vi "Calibrate NART DUT.vi"(0 "RFSA Device":refnum<k15>="RFSA" caption="instrument handle", 1 "port":u16=3363, 2 "Host":string="10.234.39.192", 3 "CART TCP Connection In":refnum<k5>, 5 "Measurement Handle In":T3, 7 "Frequency and Tx Gain":T4[](array[typedef]), 11 "error in (no error)":errorcluster, 12 "Path Loss, dB":dbl[][](array[numeric]) format="%.2f", 13 "Measurement Timeout, sec":T1=10.0 format="%.3f") -> (4 "RFSA Handle Out":T2="RFSA" caption="RFSA Handle", 6 "Measurement Handle Out":T3, 8 "CART TCP Connection Out":refnum<k5>, 15 "error out":errorcluster)   [LabVIEW 2011]
uses:
  LVx Folder/Support/TypeDef/TX Cal Data Rate.ctl
  <userlib>/niRF/niBasic/SA/Waveform/Includes/niBASIC - SA - Waveform - INC - STYP - Measurement Handle.ctl
  <userlib>/niRF/niBasic/SA/Waveform/Includes/niBASIC - SA - Waveform - INC - STYP - State Element.ctl
  <userlib>/niRF/niSystem/SA/Includes/niSYS - SA - INC - STYP - Measurement Interval.ctl
  <userlib>/niRF/niSystem/SA/Includes/niSYS - SA - INC - STYP - RBW Filter.ctl
  <userlib>/niRF/niSystem/SA/Includes/niSYS - SA - INC - STYP - External Attenuation.ctl
  <userlib>/niRF/niBasic/SA/Waveform/Includes/niBASIC - SA - Waveform - INC - STYP - Averaging.ctl
  <userlib>/niRF/niSystem/SA/Includes/niSYS - RFSA - INC - STYP - Handle.ctl
  <userlib>/niRF/niSystem/SA/Includes/niSYS - SA - INC - STYP - Timeout.ctl
  <userlib>/niRF/niSystem/SA/Includes/niSYS - SA - INC - STYP - Measurement Request.ctl
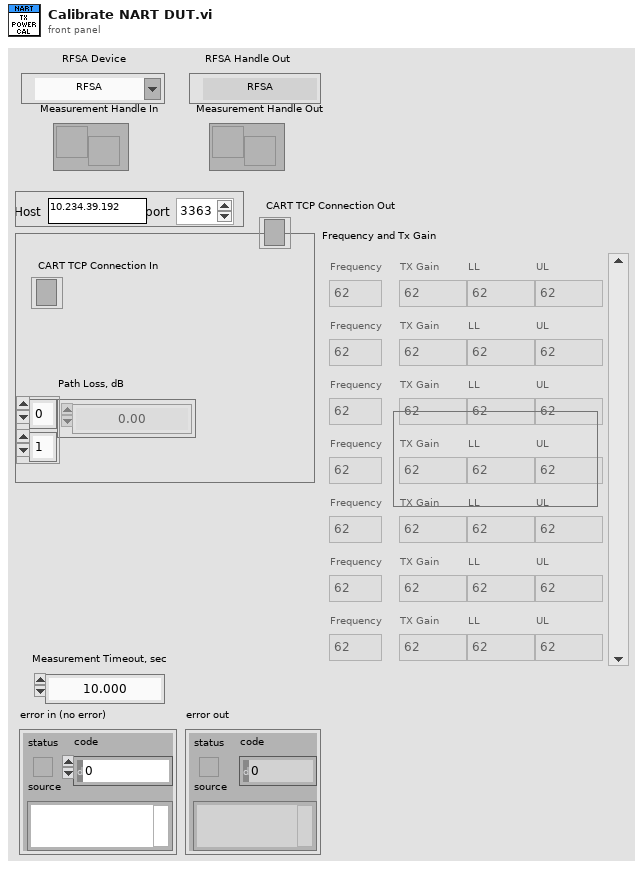
[diagram p1: front panel]
types:
  T1 = typedef "niSYS - SA - INC - STYP - Timeout.ctl" = dbl
  T2 = typedef "niSYS - RFSA - INC - STYP - Handle.ctl" = refnum<k15>
  T3 = typedef "niBASIC - SA - Waveform - INC - STYP - Measurement Handle.ctl" = refnum<notifier>
  T4 = typedef "TX Cal Data Rate.ctl" = cluster{"Frequency":u32, "TX Gain":u32, "LL":i32, "UL":u32}
  T5 = typedef "niSYS - SA - INC - STYP - Measurement Interval.ctl" = dbl
  T6 = typedef "niSYS - SA - INC - STYP - Measurement Request.ctl" = enum16{"Measure", "Fetch", "Initiate"}
  T7 = cluster{"Frequency, MHz":u32, "TX Gain":u32, "Data Rate":string, "Packet Length":u32, "Packet Count":i32}
  T8 = typedef "niBASIC - SA - Waveform - INC - STYP - Measurement.ctl" = cluster{"Mean Power, dBm":dbl, "Peak to Average Ratio, dB":dbl, "Maximum Power, dBm":dbl, "Minimum Power, dBm":dbl}
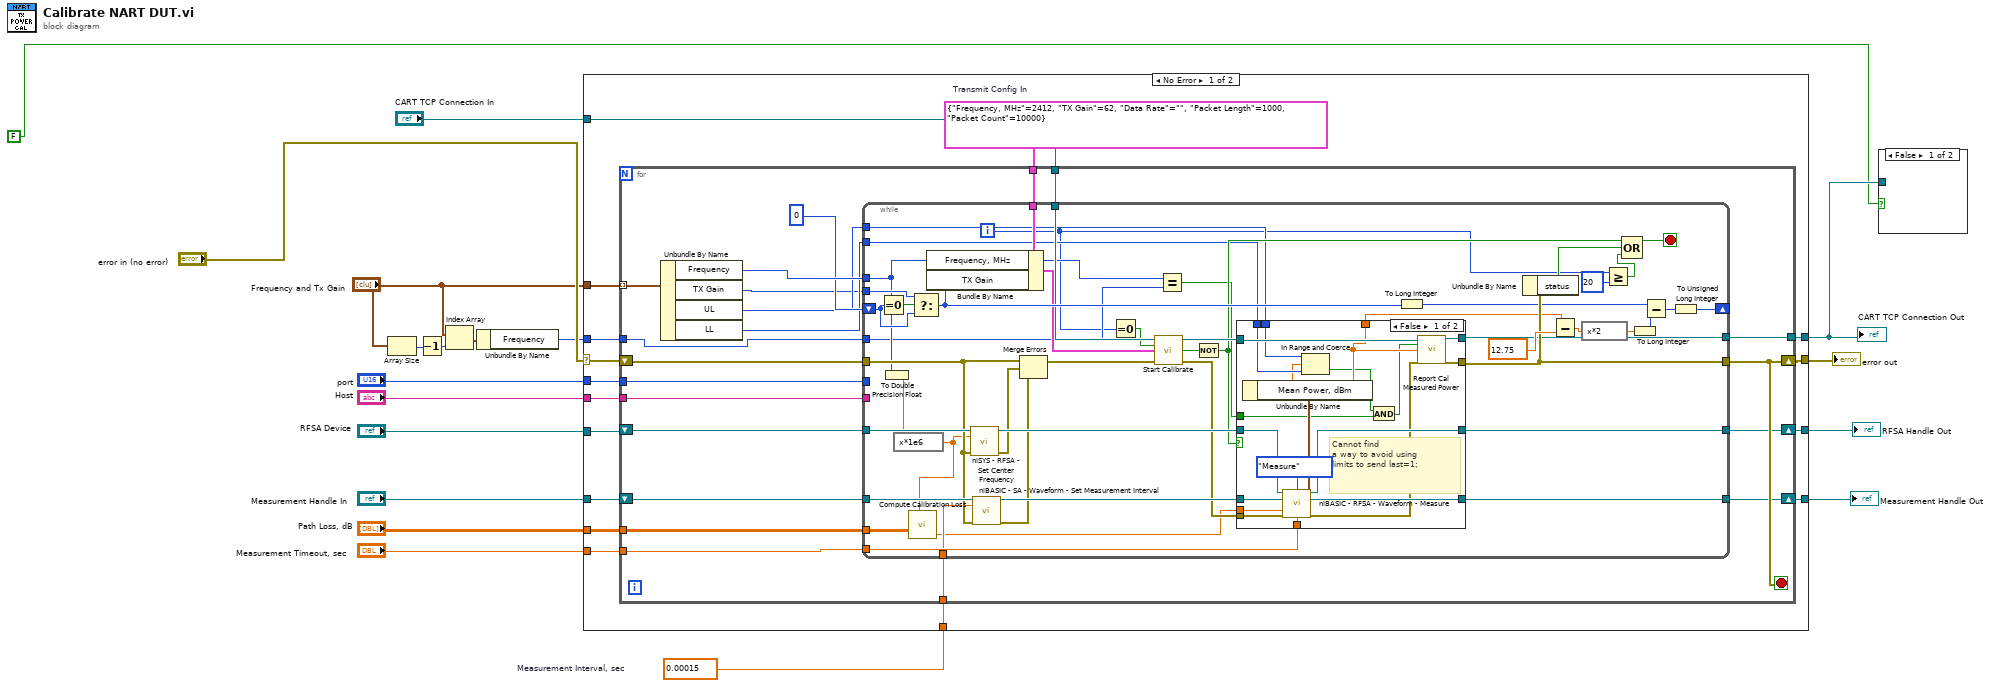
[diagram p0: block diagram]
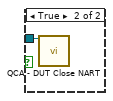
[diagram p2: hidden frame]
diagram:
  w11 = T5 0.00015  # Measurement Interval, sec
  n1 = Array Size(array="Frequency and Tx Gain") -> (size(s)=w4:i32)
  n2 = Decrement(x=w4) -> (x-1=w3:i32)
  n3 = Index Array(array="Frequency and Tx Gain", index=w3) -> (element=w2:T4)
  n4 = Unbundle By Name(w2) -> ("Frequency"=w1:u32)
  n5 = case shown="No Error" "error in (no error)" {
    selector: "error in (no error)" -> [w33 w131]
    tunnel: [w22 w131] -> w17
    tunnel: "port" -> [w21 _]
    tunnel: "Host" -> [w32 _]
    tunnel: "Frequency and Tx Gain" -> [w34 _]
    tunnel: "Measurement Handle In" -> [w31 w129]
    tunnel: [w30 w129] -> w15
    tunnel: "RFSA Device" -> [w29 w130]
    tunnel: [w28 w130] -> w13
    tunnel: "Path Loss, dB" -> [w27 _]
    tunnel: "Measurement Timeout, sec" -> [w26 _]
    tunnel: w11 -> [w25 _]
    tunnel: "CART TCP Connection In" -> [w24 w128]
    tunnel: [w20 w128] -> w9
    tunnel: w1 -> [w23 _]
    frame No Error {
      w35 = T7 {"Frequency, MHz"=2412, "TX Gain"=62, "Data Rate"="", "Packet Length"=1000, "Packet Count"=10000}  # Transmit Config In
      n6 = for {
        tunnel: w21 -> [w56]
        tunnel: w32 -> [w55]
        tunnel: w35 -> [w54]
        tunnel: w34 -> [w53] mode=indexing
        shift-right: [w52] -> w22
        shift-left: w33 -> [w51]
        shift-right: [w49] -> w30
        shift-left: w31 -> [w50]
        shift-right: [w47] -> w28
        shift-left: w29 -> [w48]
        tunnel: w27 -> [w46]
        tunnel: w26 -> [w45]
        tunnel: w25 -> [w44]
        tunnel: w24 -> [w43]
        tunnel: [w42] -> w20
        tunnel: w23 -> [w41]
        stop <- w52 stop-if-true
        n7 = Unbundle By Name(w53) -> ("Frequency"=w40:u32, "TX Gain"=w36:u32, "UL"=w38:u32, "LL"=w37:i32)
        n8 = while {
          tunnel: w54 -> [w104]
          tunnel: w56 -> [_]
          tunnel: [w78] -> w52
          tunnel: w55 -> [_]
          tunnel: w50 -> [w102]
          tunnel: [w101] -> w49
          tunnel: [w100] -> w47
          tunnel: w46 -> [w71]
          tunnel: w45 -> [w99]
          tunnel: w48 -> [w98]
          tunnel: w40 -> [w67]
          tunnel: w51 -> [w96]
          tunnel: w44 -> [w93]
          shift-right: [w84] -> _
          shift-left: u32 0 ("TX Gain") -> [w88]
          tunnel: w36 -> [w91]
          tunnel: w43 -> [w74]
          tunnel: [w72] -> w42
          tunnel: w38 -> [w62]
          tunnel: w37 -> [w61]
          tunnel: w41 -> [w66]
          i -> [w58]
          stop <- w83 stop-if-true
          n9 = Equal To 0?(x=w88) -> (x = 0?=w92:bool)
          n10 = To Double Precision Float(number=w67) -> (double precision float=w81:dbl)
          n11 = expression code="x*1e6"(w81) -> (w70:dbl)
          n12 = call "Compute Calibration Loss.vi"("Table (frequency, power, pathloss)"=w71, "Center Frequency, Hz"=w70) -> ("External Attenuation, dB"=w69:dbl)  [unwired: 3 in, 2 out]
          n13 = Select(t=w91, s=w92, f=w88) -> (s? t:f=w87:u32)
          n14 = Bundle By Name(cluster=w104, "Frequency, MHz"=w67, "TX Gain"=w87) -> (w75:T7)
          n15 = call <userlib>:"niSYS - RFSA - Set Center Frequency.vi"("RFSA Handle In"=w98, "RFSA Center Frequency, Hz"=w70, "error in (no error)"=w96) -> ("RFSA Handle Out"=w97:T2, "error out"=w95:errorcluster)  [unwired: 11 out]
          n16 = call <userlib>:"niBASIC - SA - Waveform - Set Measurement Interval.vi"("Measurement Handle In"=w102, "Measurement Interval, sec"=w93, "error in (no error)"=w96) -> ("Measurement Handle Out"=w103:T3, "error out"=w94:errorcluster)  [unwired: 11 out]
          n17 = Merge Errors(w96, w95, w94) -> (w76:errorcluster)
          n18 = Equal To 0?(x=w58) -> (x = 0?=w68:bool)
          n19 = call "Start Calibrate.vi"("CART TCP Connection In"=w74, "Send Cal Command?"=w68, "Calibrate Config"=w75, "error in (no error)"=w76) -> ("CART TCP Connection Out"=w73:refnum<k5>, "More Pwr Reporting?"=w64:bool, "error out"=w77:errorcluster)  [unwired: 7 in, 2 out]
          n20 = Equal?(x=w67, y=w66) -> (x = y?=w63:bool)
          n21 = Not(x=w64) -> (.not. x?=w65:bool)
          n22 = case shown="False" w65 {
            tunnel: w103 -> [w121 w126]
            tunnel: [w120 w126] -> w101
            tunnel: [w119 w127] -> w100
            tunnel: w99 -> [w118 _]
            tunnel: w97 -> [w117 w127]
            tunnel: [w115 w125] -> w78
            tunnel: w77 -> [w114 w125]
            tunnel: w73 -> [w113 w124]
            tunnel: [w112 w124] -> w72
            tunnel: w69 -> [w111 _]
            tunnel: [w107 _] -> w57
            tunnel: w63 -> [w110 _]
            tunnel: w62 -> [w109 _]
            tunnel: w61 -> [w108 _]
            frame False {
              # "Cannot find\na way to avoid using\nlimits to send last=1;"
              n23 = call <userlib>:"niBASIC - RFSA - Waveform - Measure.vi"("RFSA Handle In"=w117, "Measurement Request"=niSYS_-_SA_-_INC_-_STYP_-_Measurement_Request."Measure", "Measurement Handle In"=w121, "External Attenuation, dB"=w111, "error in (no error)"=w114, "Timeout, sec"=w118) -> ("RFSA Handle Out"=w119:T2, "Measurement Handle Out"=w120:T3, "Measurement"=w122:T8, "error out"=w116:errorcluster)  [unwired: 2 in, 4 out]
              n24 = Unbundle By Name(w122) -> ("Mean Power, dBm"=w107:dbl)
              n25 = In Range and Coerce(upper limit=w109, x=w107, lower limit=w108) -> (In Range?=w106:bool)  [unwired: 1 out]
              n26 = And(x=w106, y=w110) -> (x .and. y?=w105:bool)
              n27 = call "Report Cal Measured Power.vi"("CART TCP Connection In"=w113, "Commit?"=w105, "Measured Cal Power"=w107, "error in (no error)"=w116) -> ("CART TCP Connection Out"=w112:refnum<k5>, "error out"=w115:errorcluster)  [unwired: 8 in, 2 out]
            }
            frame True {
              # "Cal done for a frequency"
            }
          }
          n28 = To Long Integer(number=w87) -> (32bit integer=w60:i32)
          n29 = Unbundle By Name(w78) -> ("status"=w82:bool)
          n30 = Subtract(x=w57, y=12.75) -> (x-y=w89:dbl)
          n31 = expression code="x*2"(w89) -> (w85:dbl)
          n32 = Greater Or Equal?(x=w58, y=20) -> (x >= y?=w80:bool)
          n33 = Compound Arithmetic op=OR(w65, w82, w80) -> (w83:bool)
          n34 = To Long Integer(number=w85) -> (32bit integer=w86:i32)
          n35 = Subtract(x=w60, y=w86) -> (x-y=w59:i32)
          n36 = To Unsigned Long Integer(number=w59) -> (unsigned 32bit integer=w84:u32)
        }
      }
    }
    frame Error {
    }
  }
  "error out" <- w17
  "Measurement Handle Out" <- w15
  "RFSA Handle Out" <- w13
  "CART TCP Connection Out" <- w9
  n37 = case shown="False" FALSE {
    tunnel: w9 -> [_ w132]
    frame False {
    }
    frame True {
      n38 = call "QCA - DUT Close NART.vi"("CART TCP Connection"=w132) -> ()  [unwired: 14 in, 1 out]
    }
  }
